vi "Configure Trigger.vi"(4 "Triggered Current Limit (0.0 A)":dbl format="%.2g", 6 "Triggered Voltage Level (0.0 V)":dbl format="%.2g", 7 "Channel (1: Channel 1)":i32(ring)=1 items=["Channel 1"=1, "Channel 2"=2, "Channel 3"=3], 8 "error in (no error)":errorcluster, 9 "Trigger Delay (0 sec)":dbl min=0.0 max=3600.0 step=1.0 format="%.2f", 10 "Trigger Source (0: Immediate)":u16(ring) items=["Immediate", "Software"], 11 "VISA resource name":refnum<visa-resource-name>) -> (0 "error out":errorcluster, 3 "VISA resource name out":refnum<visa-resource-name>)   [LabVIEW 2010, in "Agilent E363X Series.lvlib"]
doc: "Configures the trigger settings on the instrument. Triggered Voltage Level and Triggered Current Limit will be set on the selected Channel when a trigger occurs."
uses:
  <instrlib>/Agilent E363X Series/Agilent E363X Series.lvlib
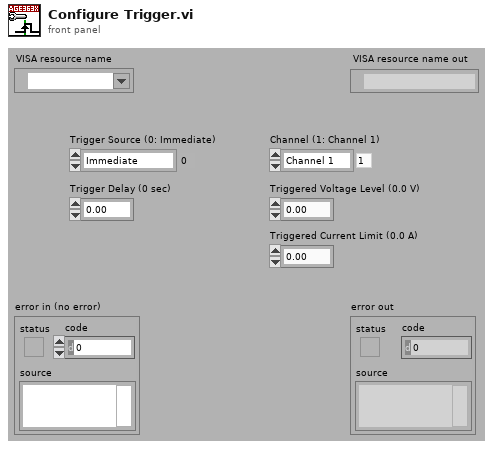
[diagram p1: front panel]
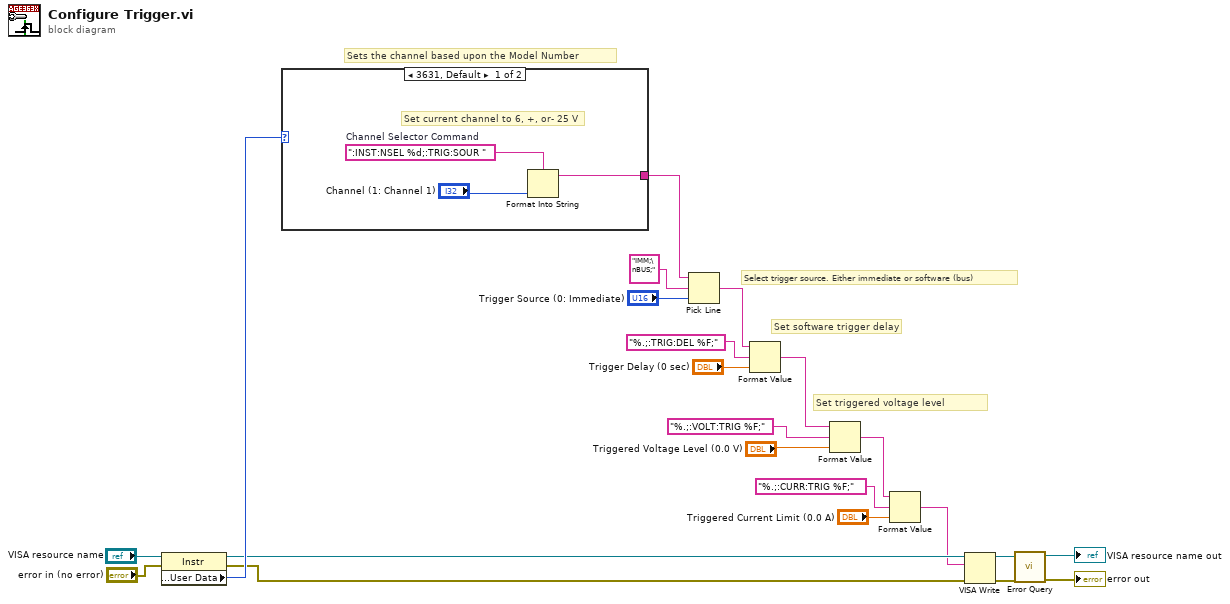
[diagram p0: block diagram]
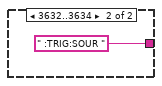
[diagram p2: hidden frame]
diagram:
  # "Set triggered voltage level"
  # "Sets the channel based upon the Model Number"
  # "Set software trigger delay"
  # "Select trigger source. Either immediate or software (bus)"
  n1 = property on="Property Node" class="Instr"(reference="VISA resource name", error in="error in (no error)") -> (reference out=w10:refnum<visa-resource-name>, error out=w9:errorcluster, "General Settings:User Data"=w13:u32)
  n2 = case shown="3631, Default" w13 {
    tunnel: [w24 " :TRIG:SOUR " ("Range Selector Command")] -> w8
    frame 3631, Default {
      w25 = ":INST:NSEL %d;:TRIG:SOUR "  # Channel Selector Command
      # "Set current channel to 6, +, or- 25 V"
      n3 = Format Into String(format string=w25, "Channel (1: Channel 1)") -> (resulting string=w24:string)  [unwired: 2 in, 1 out]
    }
    frame 3632..3634 {
    }
  }
  n4 = Pick Line(string ("")=w8, multi-line string="IMM;\nBUS;", line index="Trigger Source (0: Immediate)") -> (output string=w14:string)
  n5 = Format Value(string ("")=w14, format string="%.;:TRIG:DEL %F;", value (0)="Trigger Delay (0 sec)") -> (output string=w7:string)
  n6 = Format Value(string ("")=w7, format string="%.;:VOLT:TRIG %F;", value (0)="Triggered Voltage Level (0.0 V)") -> (output string=w4:string)
  n7 = Format Value(string ("")=w4, format string="%.;:CURR:TRIG %F;", value (0)="Triggered Current Limit (0.0 A)") -> (output string=w1:string)
  n8 = VISA Write(VISA resource name=w10, write buffer=w1, error in (no error)=w9) -> (VISA resource name out=w20:refnum<visa-resource-name>, error out=w19:errorcluster)  [unwired: 1 out]
  n9 = call <instrlib>:"Error Query.vi"("error in (no error)"=w19, "VISA resource name"=w20) -> ("error out"=→"error out":errorcluster, "VISA resource name out"=→"VISA resource name out":refnum<visa-resource-name>)  [unwired: 6 in, 2 out]
